vi "calculate_magnetization.vi"(9 "Flux constant":T1, 10 "Count":T1, 11 "Reading":T1) -> (3 "magnetization":T1)   [LabVIEW 2017]
uses:
  controls/XYZ_Data.ctl
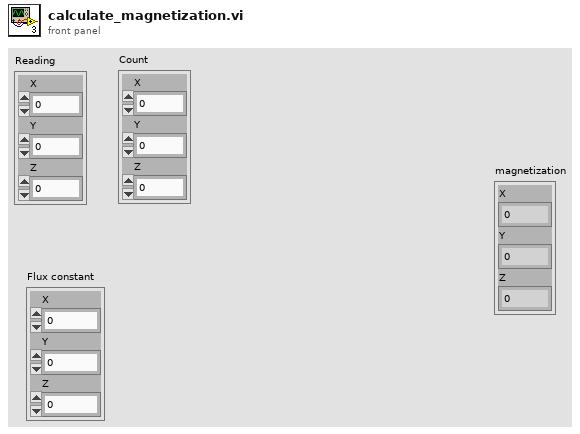
[diagram p1: front panel]
types:
  T1 = typedef "XYZ_Data.ctl" = cluster{"X":dbl, "Y":dbl, "Z":dbl}
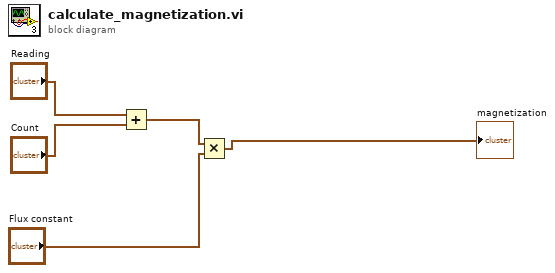
[diagram p0: block diagram]
diagram:
  n1 = Add(x="Reading", y="Count") -> (x+y=w3:T1)
  n2 = Multiply(x=w3, y="Flux constant") -> (x*y=→"magnetization":T1)
